vi "To String.vi"(11 "JSON Object in":refnum<class "JSON Object.lvclass">) -> (2 "String":string)   [LabVIEW 2017, in "LVJSON.lvlib" / "JSON Object.lvclass"]
uses:
  JSON Object.lvclass
  JSON Object.lvclass/JSON Object.ctl
  JSON Datatype/JSON Datatype.lvclass
  LVJSON.lvlib
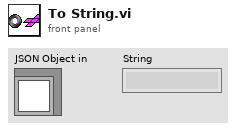
[diagram p1: front panel]
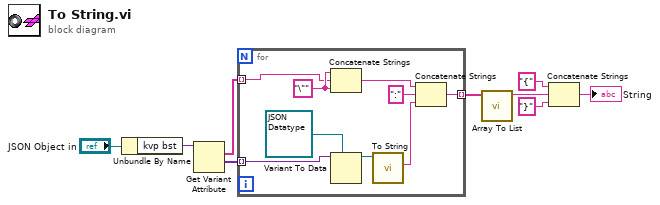
[diagram p0: block diagram]
diagram:
  n1 = Unbundle By Name("JSON Object in") -> ("kvp bst"=w8:variant)
  n2 = Get Variant Attribute(Variant=w8) -> (names=w7:string[], values=w6:variant[])  [unwired: 3 in, 2 out]
  n3 = for {
    tunnel: w7 -> [w14] mode=indexing
    tunnel: w6 -> [w18] mode=indexing
    tunnel: [w16] -> w2 mode=indexing
    w15 = "\"" ("string")
    n4 = Concatenate Strings(w15, w14, w15) -> (w13:string)
    n5 = Variant To Data(type=refnum<class "JSON Datatype.lvclass"> refnum ("JSON Datatype.lvclass"), Variant=w18) -> (data=w11:refnum<class "JSON Datatype.lvclass">)  [unwired: 1 in, 1 out]
    n6 = call-dynamic "To String.vi"("JSON Datatype in"=w11) -> ("String"=w10:string)  [unwired: 10 in]
    n7 = Concatenate Strings(w13, ":" ("string"), w10) -> (w16:string)
  }
  n8 = call "Array To List.vi"("Array"=w2) -> ("String"=w1:string)  [unwired: 10 in]
  n9 = Concatenate Strings("{" ("string"), w1, "}" ("string")) -> (→"String":string)
